vi "Load.vi"(7 "Deck ID":string, 8 "error in (no error)":errorcluster, 9 "Message Queue":refnum<queue>, 10 "Path":path, 11 "Audio Data Reference":refnum<data-value>) -> (0 "error out":errorcluster)   [LabVIEW 2018, in "Audio File Input.lvlib"]
doc: "Sets up an asynchronous call to load the audio file given in Path."
uses:
  Audio File Input.lvlib
  Messaging/Message Cluster.ctl
  Messaging/Messaging.lvlib
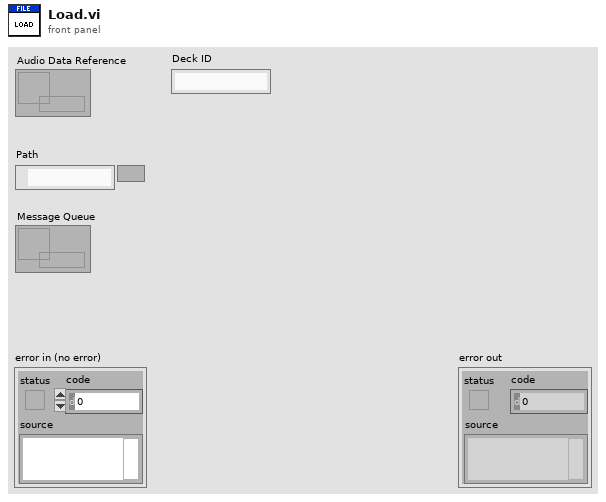
[diagram p1: front panel]
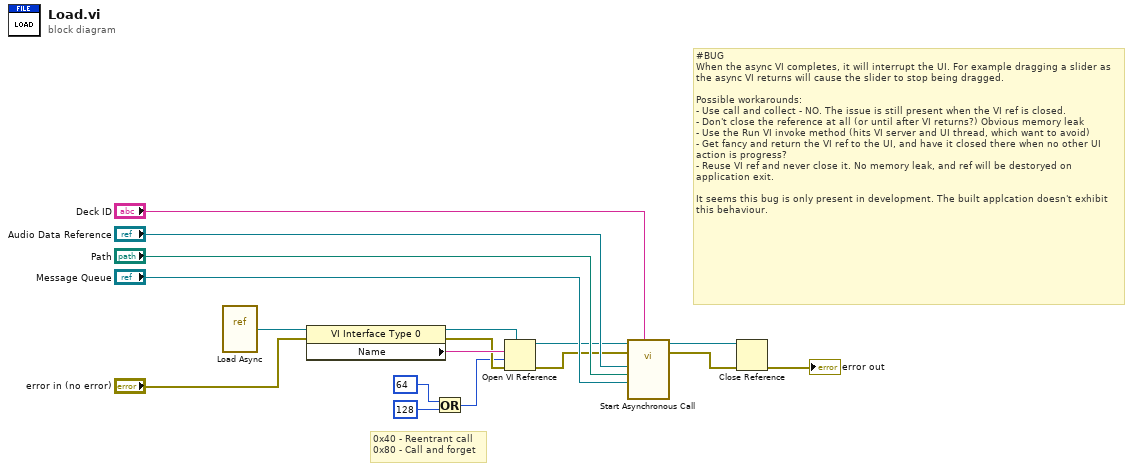
[diagram p0: block diagram]
diagram:
  # "0x40 - Reentrant call\n0x80 - Call and forget"
  # "#BUG\nWhen the async VI completes, it will interrupt the UI. For example dragging a slider as the async VI returns will cause the slider to stop being dragged.\n\nPossible workarounds:\n- Use call and collect - NO. The issue is still present when the VI ref is closed.\n- Don't close the reference at all (or until after VI returns?) Obvious memory leak\n- Use the Run VI invoke method (hits VI server and UI thread, which want to avoid)\n- Get fancy and return the VI ref to the UI, and have it closed there when no other UI action is progress?\n- Reuse VI ref and never close it. No memory leak, and ref will be destoryed on application exit.\n\nIt seems this bug is only present in development. The built applcation doesn't exhibit this behaviour."
  n1 = vi-ref "Load Async.vi"() -> (w7:refnum<vi>)
  n2 = property class="VI Interface Type 0"(reference=w7, error in="error in (no error)") -> (reference out=w1:refnum<vi>, error out=w5:errorcluster, "Name"=w6:string)
  n3 = Or(x=64 ("options"), y=128 ("options")) -> (x .or. y?=w2:i32)
  n4 = Open VI Reference(type specifier VI Refnum (for type only)=w1, vi path=w6, options=w2, error in (no error)=w5) -> (vi reference=w11:refnum<vi>, error out=w10:errorcluster)  [unwired: 2 in]
  n5 = call-by-ref "Start Asynchronous Call"(reference=w11, error in=w10, "Deck ID"="Deck ID", "Message Queue"="Message Queue", "Path"="Path", "Audio Data Reference"="Audio Data Reference") -> (reference out=w8:refnum<vi>, error out=w9:errorcluster)  [unwired: 7 in, 1 out]
  n6 = Close Reference(reference=w8, error in (no error)=w9) -> (error out=→"error out":errorcluster)
